vi "QMH_QRef.vi"(6 "Get/Set (Get=F)":bool, 7 "Enum":T1, 8 "error in (no error)":errorcluster, 11 "Cluster In":T2) -> (0 "error out":errorcluster, 2 "Queue_ref":refnum<queue>, 3 "Cluster Out":T2)   [LabVIEW 2021, in "Framework_lib.lvlib"]
uses:
  Framework_lib.lvlib
  QMH_references.ctl
  framework_Qmessage.ctl
  QMH_producer_enum.ctl
  QMH_references_enum.ctl
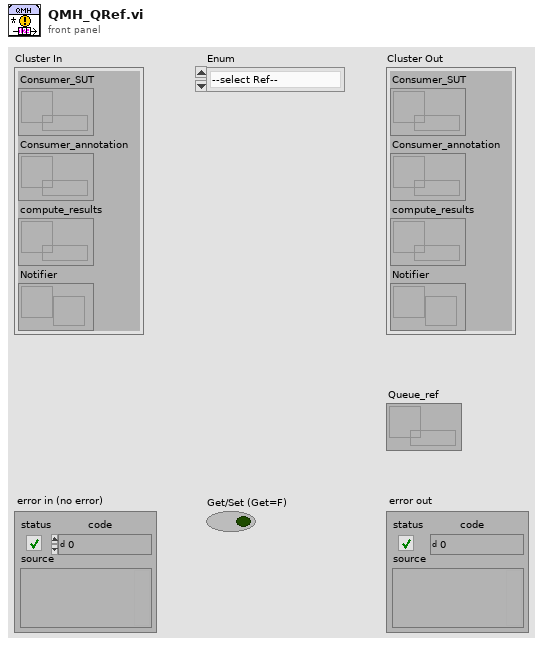
[diagram p1: front panel]
types:
  T1 = typedef "Framework_lib.lvlib/QMH_references_enum.ctl" = enum16{"--select Ref--", "Consumer_SUT", "Consumer_Annot", "Compute_Results"}
  T2 = typedef "Framework_lib.lvlib/QMH_references.ctl" = cluster{"Consumer_SUT":refnum<queue>, "Consumer_annotation":refnum<queue>, "compute_results":refnum<queue>, "Notifier":refnum<notifier>}
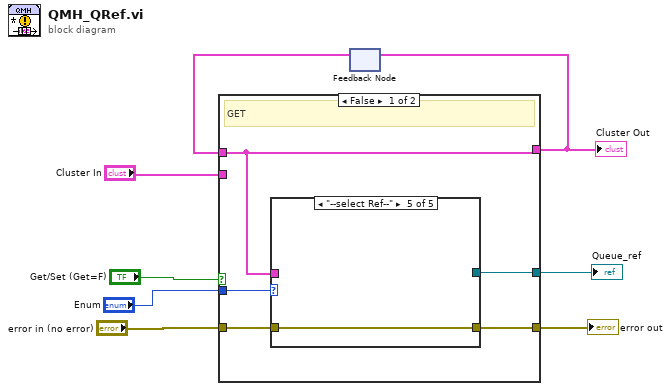
[diagram p0: block diagram]
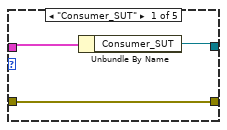
[diagram p2: hidden frame]
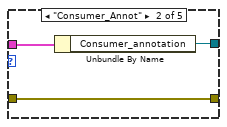
[diagram p3: hidden frame]
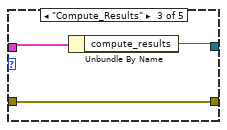
[diagram p4: hidden frame]
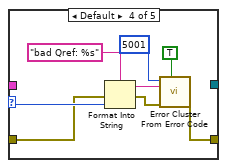
[diagram p5: hidden frame]
diagram:
  n1 = feedback #1() -> (w7:T2)  [unwired: 1 in]
  n2 = case shown="False" "Get/Set (Get=F)" {
    tunnel: "Cluster In" -> [_ w33]
    tunnel: w7 -> [w13 _]
    tunnel: [w13 w33] -> w1
    tunnel: "Enum" -> [w12 _]
    tunnel: "error in (no error)" -> [w11 w32]
    tunnel: [w10 _] -> w3
    tunnel: [w9 w32] -> w2
    frame False {
      # "GET"
      n3 = case shown="\"--select Ref--\"" w12 {
        selector: w12 -> [_ _ _ w30 _]
        tunnel: w13 -> [w15 w19 w21 _ _]
        tunnel: [w16 w18 w22 _ _] -> w10
        tunnel: w11 -> [w14 w17 w20 w24 w31]
        tunnel: [w14 w17 w20 w25 w31] -> w9
        frame "Consumer_SUT" {
          n4 = Unbundle By Name(w15) -> ("Consumer_SUT"=w16:refnum<queue>)
        }
        frame "Consumer_Annot" {
          n5 = Unbundle By Name(w19) -> ("Consumer_annotation"=w18:refnum<queue>)
        }
        frame "Compute_Results" {
          n6 = Unbundle By Name(w21) -> ("compute_results"=w22:refnum<queue>)
        }
        frame Default {
          n7 = Format Into String(format string="bad Qref: %s", error in=w24, w30) -> (resulting string=w27:string, error out=w28:errorcluster)  [unwired: 1 in]
          n8 = call <vilib>:"Error Cluster From Error Code.vi"("show call chain? (False)"=TRUE, "error in (no error)"=w28, "error message (\"\")"=w27, "error code (0)"=5001) -> ("error out"=w25:errorcluster)  [unwired: 5 in]
        }
        frame "--select Ref--" {
        }
      }
    }
    frame True {
      # "SET"
    }
  }
  "error out" <- w2
  "Cluster Out" <- w1
  "Queue_ref" <- w3
  n9 = feedback-in #1(w1) -> ()
